vi "FT Write GPIO.vi"(5 "value":u8, 7 "dir":u8, 8 "error in (no error)":errorcluster, 11 "handle":u32) -> (0 "error out":errorcluster, 3 "handle out":u32)   [LabVIEW 2018, in "libMPSSE-SPI.lvlib"]
doc: "FTDI_API FT_STATUS FT_WriteGPIO(FT_HANDLE handle, uint8 dir, uint8 value);"
uses:
  libMPSSE-SPI.lvlib
  dll/libMPSSE.dll
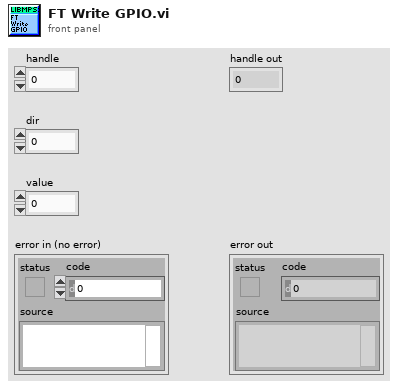
[diagram p1: front panel]
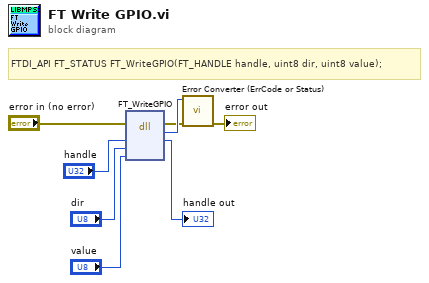
[diagram p0: block diagram]
diagram:
  # "FTDI_API FT_STATUS FT_WriteGPIO(FT_HANDLE handle, uint8 dir, uint8 value);"
  n1 = dll-call lib="D:/LABVIEW/Examples - 32bit/FTDI/libMPSSE-SPI-LabVIEW-master/dll/libMPSSE.*" fn="FT_WriteGPIO"(error in="error in (no error)", "handle"="handle", "dir"="dir", "value"="value") -> (error out=w2:errorcluster, "return type"=w8:u32, "handle"=→"handle out":u32)  [unwired: 4 in, 1 out]
  n2 = call "Error Converter (ErrCode or Status).vi"("error in (no error)"=w2, "error code"=w8) -> ("error out"=→"error out":errorcluster)  [unwired: 9 in]
